vi "FOCUS_V42_H37.vi"(9 "X-pixels":sgl=256.0, 11 "Run":bool) -> (0 "Retrace pixels":sgl, 10 "Pixel Clock (Hz)":sgl)   [LabVIEW 2010] (continued)
                    n2567 = local read "stop 2"() -> (w4781:bool)
                    n2568 = Increment(x=w4763) -> (x+1=w4798:i32)
                    "#" <- w4798
                    n2569 = local read "Overlay Images"() -> (w4802:bool)
                    n2570 = Array Subset "Extract DI0"(array=w4764, index=w4789, length=w4791) -> (w4794:u32[])
                    n2571 = Equal?(x=w4798, y=w4777) -> (x = y?=w4779:bool)
                    n2572 = Split Number(x=w4794) -> (hi(x)=w4753:u16[], lo(x)=w4761:u16[])
                    n2573 = case shown="0, Default" w4760 {
                      tunnel: w4753 -> [w4829 w4834 w4839 w4844 w4849 w4854]
                      tunnel: [w4828 w4833 w4836 w4843 w4848 w4851] -> w4758
                      tunnel: [w4826 w4831 w4838 w4841 w4846 w4853] -> w4757
                      tunnel: w4761 -> [w4827 w4832 w4837 w4842 w4847 w4852]
                      tunnel: [w4825 w4830 w4835 w4840 w4845 w4850] -> w4759
                      frame 0, Default {
                        n2574 = Split Number(x=w4829) -> (hi(x)=w4828:u8[], lo(x)=w4826:u8[])
                        n2575 = Split Number(x=w4827) -> (lo(x)=w4825:u8[])  [unwired: 1 out]
                      }
                      frame 1 {
                        n2576 = Split Number(x=w4834) -> (hi(x)=w4833:u8[], lo(x)=w4830:u8[])
                        n2577 = Split Number(x=w4832) -> (lo(x)=w4831:u8[])  [unwired: 1 out]
                      }
                      frame 2 {
                        n2578 = Split Number(x=w4839) -> (hi(x)=w4835:u8[], lo(x)=w4838:u8[])
                        n2579 = Split Number(x=w4837) -> (lo(x)=w4836:u8[])  [unwired: 1 out]
                      }
                      frame 3 {
                        n2580 = Split Number(x=w4844) -> (hi(x)=w4843:u8[], lo(x)=w4841:u8[])
                        n2581 = Split Number(x=w4842) -> (lo(x)=w4840:u8[])  [unwired: 1 out]
                      }
                      frame 4 {
                        n2582 = Split Number(x=w4849) -> (hi(x)=w4848:u8[], lo(x)=w4845:u8[])
                        n2583 = Split Number(x=w4847) -> (lo(x)=w4846:u8[])  [unwired: 1 out]
                      }
                      frame 5 {
                        n2584 = Split Number(x=w4854) -> (hi(x)=w4850:u8[], lo(x)=w4853:u8[])
                        n2585 = Split Number(x=w4852) -> (lo(x)=w4851:u8[])  [unwired: 1 out]
                      }
                    }
                    n2586 = Set File Position(refnum=w4775, from (0:start)=enum16{"start", "end", "current"}."current" ("pos mode (0:2)"), error in=w4774) -> (refnum out=w4750:refnum<file>, error out=w4749:errorcluster)  [unwired: 1 in]
                    n2587 = Compound Arithmetic op=OR(w4779, w4780, w4781, w4783, w4782, w4784, w4785) -> (w4778:bool)
                    n2588 = Tick Count (ms)() -> (millisecond timer value=w4810:u32)
                    n2589 = case shown="1" w4762 {
                      tunnel: w4758 -> [w4857 w4865]
                      tunnel: [w4857 w4864] -> w4756
                      tunnel: w4763 -> [_ w4860]
                      tunnel: w4757 -> [w4856 w4862]
                      tunnel: [w4856 w4861] -> w4755
                      tunnel: w4759 -> [w4855 w4859]
                      tunnel: [w4855 w4858] -> w4754
                      frame 0, Default {
                      }
                      frame 1 {
                        n2590 = local read "Shift"() -> (w4863:sgl)
                        n2591 = call "testoddevenFOCUS.vi"("Numeric"=w4860) -> ("Boolean"=w4866:bool)
                        n2592 = case shown="True" w4866 {
                          tunnel: w4865 -> [w4869 w4896]
                          tunnel: [w4869 w4898] -> w4864
                          tunnel: w4863 -> [_ w4872]
                          tunnel: w4862 -> [w4868 w4884]
                          tunnel: [w4868 w4883] -> w4861
                          tunnel: w4859 -> [w4867 w4871]
                          tunnel: [w4867 w4870] -> w4858
                          frame False {
                          }
                          frame True {
                            n2593 = Round Toward -Infinity(1:w4872) -> (0:w4888:sgl)
                            n2594 = Round Toward -Infinity(1:w4872) -> (0:w4879:sgl)
                            n2595 = Round Toward -Infinity(1:w4872) -> (0:w4903:sgl)
                            n2596 = To Word Integer(number=w4884) -> (16bit integer=w4894:i16[])
                            n2597 = To Word Integer(number=w4871) -> (16bit integer=w4873:i16[])
                            n2598 = To Word Integer(number=w4896) -> (16bit integer=w4895:i16[])
                            n2599 = Array Subset(array=w4894, index=1) -> (w4887:i16[])  [unwired: 1 in]
                            n2600 = Array Subset(array=w4873, index=1) -> (w4880:i16[])  [unwired: 1 in]
                            n2601 = Array Subset(array=w4895, index=1) -> (w4904:i16[])  [unwired: 1 in]
                            n2602 = Subtract(x=w4872, y=w4888) -> (x-y=w4889:sgl)
                            n2603 = Subtract(x=w4872, y=w4879) -> (x-y=w4878:sgl)
                            n2604 = Subtract(x=w4872, y=w4903) -> (x-y=w4902:sgl)
                            n2605 = Subtract(x=w4894, y=w4887) -> (x-y=w4891:i16[])
                            n2606 = Subtract(x=w4873, y=w4880) -> (x-y=w4876:i16[])
                            n2607 = Subtract(x=w4895, y=w4904) -> (x-y=w4900:i16[])
                            n2608 = Build Array (concatenate)(0 ("index"), w4891) -> (w4892:i32[])
                            n2609 = Build Array (concatenate)(0 ("index"), w4876) -> (w4875:i32[])
                            n2610 = Build Array (concatenate)(0 ("index"), w4900) -> (w4899:i32[])
                            n2611 = Multiply(x=w4889, y=w4892) -> (x*y=w4890:sgl[])
                            n2612 = Multiply(x=w4878, y=w4875) -> (x*y=w4877:sgl[])
                            n2613 = Multiply(x=w4902, y=w4899) -> (x*y=w4901:sgl[])
                            n2614 = Add(x=w4894, y=w4890) -> (x+y=w4885:sgl[])
                            n2615 = To Unsigned Byte Integer(number=w4885) -> (unsigned 8bit integer=w4883:u8[])
                            n2616 = Add(x=w4873, y=w4877) -> (x+y=w4882:sgl[])
                            n2617 = To Unsigned Byte Integer(number=w4882) -> (unsigned 8bit integer=w4870:u8[])
                            n2618 = Add(x=w4895, y=w4901) -> (x+y=w4906:sgl[])
                            n2619 = To Unsigned Byte Integer(number=w4906) -> (unsigned 8bit integer=w4898:u8[])
                          }
                        }
                      }
                    }
                    n2620 = case shown="True" w4802 {
                      tunnel: w4756 -> [w4926 w4929]
                      tunnel: [w4926 w4927] -> w4804
                      tunnel: w4755 -> [w4925 w4928]
                      tunnel: [w4925 _] -> w4803
                      frame False {
                      }
                      frame True {
                        n2621 = To Word Integer(number=w4929) -> (16bit integer=w4934:i16[])
                        n2622 = Subtract(x=w4934, y=w4928) -> (x-y=w4935:i16[])
                        n2623 = Add(x=w4934, y=w4928) -> (x+y=w4939:i16[])
                        n2624 = Increment(x=w4939) -> (x+1=w4930:i16[])
                        n2625 = Divide(x=w4935, y=w4930) -> (x/y=w4931:dbl[])
                        n2626 = Absolute Value(x=w4935) -> (abs(x)=w4937:i16[])
                        n2627 = Multiply(x=w4931, y=u8 2) -> (x*y=w4933:dbl[])
                        n2628 = Round To Nearest(number=w4933) -> (nearest integer value=w4946:dbl[])
                        n2629 = Divide(x=w4937, y=2.0) -> (x/y=w4940:dbl[])
                        n2630 = Divide(x=w4939, y=2.0) -> (x/y=w4941:dbl[])
                        n2631 = Add(x=w4940, y=w4941) -> (x+y=w4943:dbl[])
                        n2632 = Divide(x=w4943, y=5.0) -> (x/y=w4944:dbl[])
                        n2633 = Round To Nearest(number=w4944) -> (nearest integer value=w4945:dbl[])
                        n2634 = Multiply(x=5.0 ("y"), y=w4945) -> (x*y=w4947:dbl[])
                        n2635 = Add(x=w4946, y=w4947) -> (x+y=w4948:dbl[])
                        n2636 = Subtract(x=w4948, y=2.0) -> (x-y=w4951:dbl[])
                        n2637 = To Unsigned Byte Integer(number=w4951) -> (unsigned 8bit integer=w4927:u8[])
                      }
                    }
                    n2638 = Subtract(x=w4763, y=w4791) -> (x-y=w4792:sgl)
                    n2639 = Subtract(x=w4810, y=w4809) -> (x-y=w4811:u32)
                    n2640 = local read "Image Update [ms]"() -> (w4793:u32)
                    n2641 = property class="DAQmx Read"(reference=w4771, error in=w4769) -> (reference out=w4770:refnum<k21>, error out=w4768:errorcluster, "Status:Available Samples Per Channel"=w4767:u32)
                    n2642 = Greater Or Equal?(x=w4811, y=w4793) -> (x >= y?=w4812:bool)
                    n2643 = local write "Scan Backlock"(w4767) -> ()
                    n2644 = case shown="True" w4751 {
                      tunnel: w4756 -> [w4821 w4824]
                      tunnel: w4755 -> [w4818 w4823]
                      tunnel: w4754 -> [w4820 _]
                      tunnel: [w4819 w4822] -> w4752
                      frame True {
                        n2645 = Interleave 1D Arrays(w4818, w4821, w4820) -> (w4819:u8[])
                      }
                      frame False {
                        n2646 = Interleave 1D Arrays(w4824, w4823) -> (w4822:u8[])
                      }
                    }
                    n2647 = Write to Binary File(file (use dialog)=w4750, data=w4752, error in=w4749, 5:FALSE ("prepend array or string size? (T)")) -> (refnum out=w4773:refnum<file>, error out=w4772:errorcluster)  [unwired: 2 in, 1 out]
                    n2648 = local read "X-pixels"() -> (w4813:sgl)
                    n2649 = Subtract(x=w4763, y=w4813) -> (x-y=w4805:sgl)
                    n2650 = Replace Array Subset(array=w4817, new element=w4804, index (col)=w4763) -> (w4815:u8[][])  [unwired: 1 in]
                    n2651 = Replace Array Subset(array=w4816, new element=w4803, index (col)=w4763) -> (w4814:u8[][])  [unwired: 1 in]
                    n2652 = Array Subset(array=w4815, index (col)=w4805, length (col)=w4813) -> (w4807:u8[][])  [unwired: 2 in]
                    n2653 = Array Subset(array=w4814, index (col)=w4805, length (col)=w4813) -> (w4806:u8[][])  [unwired: 2 in]
                    n2654 = case shown="True" w4812 {
                      tunnel: [w4952 w4955] -> w4808
                      tunnel: w4809 -> [w4952 _]
                      tunnel: w4807 -> [_ w4954]
                      tunnel: w4806 -> [_ w4953]
                      frame False {
                      }
                      frame True {
                        n2655 = local write "Image 2"(w4953) -> ()
                        n2656 = local write "Image 1"(w4954) -> ()
                        n2657 = Tick Count (ms)() -> (millisecond timer value=w4955:u32)
                      }
                    }
                  }
                  n2658 = Close File(refnum=w4699, error in=w4700) -> ()  [unwired: 2 out]
                  n2659 = flat-sequence {
                    tunnel: w4732 -> [w4746]
                    tunnel: [w4746] -> w4731
                    frame #0 {
                      n2660 = Tick Count (ms)() -> (millisecond timer value=w4747:u32)
                      n2661 = local write "stop"(w4747) -> ()
                    }
                  }
                }
                frame 3 {
                  w5005 = 0.0 ("X Scale.Range:Minimum")
                  w5018 = 0.0 ("x offset")
                  w5019 = 1.0 ("x offset")
                  w5007 = TRUE ("Visible")
                  # "User-defined line"
                  n2662 = property on="Property Node" class="VI"() -> ("VI Path"=w4973:path)  [unwired: 2 in, 2 out]
                  n2663 = flat-sequence {
                    tunnel: w5012 -> [w5034]
                    tunnel: [w5034] -> w5011
                    frame #0 {
                      n2664 = Tick Count (ms)() -> (millisecond timer value=w5035:u32)
                      n2665 = local write "start"(w5035) -> ()
                    }
                  }
                  n2666 = Greater Or Equal?(x=w4961, y=u16 3) -> (x >= y?=w4959:bool)
                  n2667 = Strip Path(path=w4973) -> (stripped path=w4972:path)  [unwired: 1 out]
                  n2668 = Tick Count (ms)() -> (millisecond timer value=w5025:u32)
                  n2669 = Bundle("x offset"=w5019, "x offset"=w5019, "x offset"=w5018, "x offset"=w5018) -> (w5017:T33)  [unwired: 1 in]
                  n2670 = Build Path(base path=w4972, name or relative path="FreeLine.tmp") -> (appended path=w4971:path)
                  n2671 = Unbundle By Name(w4987) -> ("status"=w4986:bool)
                  n2672 = call <vilib>:"Open_Create_Replace File.vi"("advisory dialog? (display:T)"=FALSE, "function (open:0)"=T8."create or replace", "file path"=w4971) -> ("error out"=w4965:errorcluster, "refnum"=w4967:refnum<file>)  [unwired: 5 in, 2 out]
                  n2673 = Set File Position(refnum=w4967, from (0:start)=enum16{"start", "end", "current"}."start" ("pos mode (rel. to end:1)"), error in=w4965) -> (refnum out=w4958:refnum<file>, error out=w4957:errorcluster)  [unwired: 1 in]
                  n2674 = Write to Binary File(file (use dialog)=w4958, data=w4963, error in=w4957, 5:FALSE ("prepend array or string size? (T)")) -> (refnum out=w4966:refnum<file>, error out=w4964:errorcluster)  [unwired: 2 in, 1 out]
                  n2675 = while {
                    tunnel: [w5055] -> w5026
                    tunnel: [w5056] -> w5010
                    tunnel: w5027 -> [w5101]
                    tunnel: w5011 -> [w5100]
                    shift-right: [w5116] -> w4979
                    shift-left: w5028 -> [w5142]
                    tunnel: w4989 -> [w5098]
                    shift-right: [w5117] -> w4978
                    shift-left: w5028 -> [w5141]
                    shift-right: [w5135] -> _
                    shift-left: w5025 -> [w5136]
                    tunnel: w5023 -> [w5127]
                    tunnel: w5022 -> [w5091]
                    tunnel: [w5126] -> w5021
                    tunnel: [w5125] -> w5020
                    shift-right: [w5122] -> _
                    shift-left: w5017 -> [w5129]
                    tunnel: w5016 -> [w5104]
                    tunnel: w5015 -> [w5092]
                    tunnel: [w5103] -> w5014
                    tunnel: [w5102] -> w5013
                    shift-right: [w5107] -> w4969
                    shift-left: w5003 -> [w5109]
                    tunnel: w4993 -> [w5105]
                    tunnel: w4992 -> [w5083]
                    tunnel: [w5105] -> w4991
                    tunnel: [w5083] -> w4990
                    tunnel: [w5095] -> w4988
                    tunnel: w4986 -> [w5090]
                    shift-right: [w5059] -> w4977
                    shift-left: w4966 -> [w5062]
                    shift-right: [w5060] -> w4976
                    shift-left: w4964 -> [w5061]
                    tunnel: w4962 -> [w5053]
                    tunnel: w4961 -> [w5045]
                    tunnel: w4959 -> [w5039]
                    i -> [w5094]
                    stop <- w5081 stop-if-true
                    # "DIO Read reads one\nline of data at a time"
                    n2676 = Equal To 0?(x=w5094) -> (x = 0?=w5113:bool)
                    n2677 = local read "End experiment"() -> (w5088:bool)
                    n2678 = case shown="True" w5113 {
                      tunnel: w5098 -> [w5208 w5211]
                      tunnel: [w5208 w5210] -> w5050
                      tunnel: w5053 -> [_ w5209]
                      tunnel: [sgl 0.0 w5209] -> w5049
                      frame False {
                      }
                      frame True {
                        n2679 = Add(x=w5211, y=w5209) -> (x+y=w5210:sgl)
                      }
                    }
                    n2680 = call-poly <vilib>:"DAQmx Read (Digital 1D U32 1Chan NSamp).vi"("task/channels in"=w5101, "number of samples per channel"=w5050, "error in"=w5100) -> ("task out"=w5058:refnum<k21>, "data"=w5052:u32[], "error out"=w5057:errorcluster)  [unwired: 10 in]
                    n2681 = Increment(x=w5094) -> (x+1=w5106:i32)
                    "#" <- w5106
                    n2682 = call-poly <vilib>:"DAQmx Read (Analog 2D DBL NChan NSamp).vi"("task/channels in"=w5104, "number of samples per channel"=w5050, "error in"=w5092) -> ("task out"=w5103:refnum<k21>, "data"=w5048:dbl[][], "error out"=w5102:errorcluster)  [unwired: 10 in]
                    n2683 = Unbundle By Name(w5092) -> ("status"=w5082:bool)
                    n2684 = local read "stop 2"() -> (w5089:bool)
                    n2685 = local read "Overlay Images"() -> (w5110:bool)
                    n2686 = Array Subset(array=w5048, index (col)=w5049) -> (w5047:dbl[][])  [unwired: 3 in]
                    n2687 = Unbundle By Name(w5091) -> ("status"=w5084:bool)
                    n2688 = Equal?(x=w5106, y="Y-lines FreeLine") -> (x = y?=w5087:bool)
                    n2689 = Transpose 2D Array(2D array=w5047) -> (transposed array=w5099:dbl[][])
                    n2690 = Unbundle By Name(w5057) -> ("status"=w5085:bool)
                    n2691 = Array Subset "Extract DI0"(array=w5052, index=w5049) -> (w5051:u32[])  [unwired: 1 in]
                    n2692 = Unbundle By Name(w5083) -> ("status"=w5086:bool)
                    n2693 = Split Number(x=w5051) -> (hi(x)=w5041:u16[], lo(x)=w5046:u16[])
                    n2694 = Build Array (concatenate)(w5109, w5099) -> (w5108:dbl[][])
                    n2695 = Index Array(array=w5099, index (col)=0 ("disabled index (col)")) -> (element=w5119:dbl[])  [unwired: 1 in]
                    n2696 = Bundle("x offset"="x offset", "x scale"="x scale", "y offset"="y offset", "y scale"="y scale") -> (w5122:T34)  [unwired: 1 in]
                    n2697 = Array Subset(array=w5108, index (row)=w5098) -> (w5107:dbl[][])  [unwired: 3 in]
                    n2698 = Index Array(array=w5099, index (col)=1 ("disabled index (col)")) -> (element=w5118:dbl[])  [unwired: 1 in]
                    n2699 = Tick Count (ms)() -> (millisecond timer value=w5137:u32)
                    n2700 = Not Equal?(x=w5129, y=w5122) -> (x != y?=w5128:bool)
                    n2701 = Compound Arithmetic op=OR(w5082, w5084, w5085, w5086, w5087, w5088, w5089, w5090) -> (w5081:bool)
                    n2702 = case shown="True" w5128 {
                      tunnel: w5127 -> [w5213 w5218]
                      tunnel: w5091 -> [w5212 w5215]
                      tunnel: [w5213 w5216] -> w5126
                      tunnel: [w5212 w5214] -> w5125
                      tunnel: w5122 -> [_ w5220]
                      frame False {
                      }
                      frame True {
                        n2703 = local read "ScanLineFreeLine"() -> (w5219:sgl[][])
                        n2704 = call "ScaleudlFOCUS.vi"("Cluster"=w5220, "ScanLineUDL"=w5219) -> ("ScanLineUDLnew"=w5217:dbl[][])
                        n2705 = call-poly <vilib>:"DAQmx Write (Analog 2D DBL NChan NSamp).vi"("task/channels in"=w5218, "data"=w5217, "error in"=w5215) -> ("task out"=w5216:refnum<k21>, "error out"=w5214:errorcluster)  [unwired: 10 in, 1 out]
                      }
                    }
                    n2706 = case shown="0, Default" w5045 {
                      tunnel: w5041 -> [w5154 w5159 w5164 w5169 w5174 w5179]
                      tunnel: [w5153 w5158 w5161 w5168 w5173 w5176] -> w5042
                      tunnel: [w5151 w5156 w5163 w5166 w5171 w5178] -> w5043
                      tunnel: w5046 -> [w5152 w5157 w5162 w5167 w5172 w5177]
                      tunnel: [w5150 w5155 w5160 w5165 w5170 w5175] -> w5044
                      frame 0, Default {
                        n2707 = Split Number(x=w5154) -> (hi(x)=w5153:u8[], lo(x)=w5151:u8[])
                        n2708 = Split Number(x=w5152) -> (lo(x)=w5150:u8[])  [unwired: 1 out]
                      }
                      frame 1 {
                        n2709 = Split Number(x=w5159) -> (hi(x)=w5158:u8[], lo(x)=w5155:u8[])
                        n2710 = Split Number(x=w5157) -> (lo(x)=w5156:u8[])  [unwired: 1 out]
                      }
                      frame 2 {
                        n2711 = Split Number(x=w5164) -> (hi(x)=w5160:u8[], lo(x)=w5163:u8[])
                        n2712 = Split Number(x=w5162) -> (lo(x)=w5161:u8[])  [unwired: 1 out]
                      }
                      frame 3 {
                        n2713 = Split Number(x=w5169) -> (hi(x)=w5168:u8[], lo(x)=w5166:u8[])
                        n2714 = Split Number(x=w5167) -> (lo(x)=w5165:u8[])  [unwired: 1 out]
                      }
                      frame 4 {
                        n2715 = Split Number(x=w5174) -> (hi(x)=w5173:u8[], lo(x)=w5170:u8[])
                        n2716 = Split Number(x=w5172) -> (lo(x)=w5171:u8[])  [unwired: 1 out]
                      }
                      frame 5 {
                        n2717 = Split Number(x=w5179) -> (hi(x)=w5175:u8[], lo(x)=w5178:u8[])
                        n2718 = Split Number(x=w5177) -> (lo(x)=w5176:u8[])  [unwired: 1 out]
                      }
                    }
                    n2719 = case shown="True" w5110 {
                      tunnel: w5042 -> [w5181 w5184]
                      tunnel: [w5181 w5182] -> w5112
                      tunnel: w5043 -> [w5180 w5183]
                      tunnel: [w5180 _] -> w5111
                      frame False {
                      }
                      frame True {
                        n2720 = To Word Integer(number=w5184) -> (16bit integer=w5189:i16[])
                        n2721 = Subtract(x=w5189, y=w5183) -> (x-y=w5190:i16[])
                        n2722 = Add(x=w5189, y=w5183) -> (x+y=w5194:i16[])
                        n2723 = Increment(x=w5194) -> (x+1=w5185:i16[])
                        n2724 = Divide(x=w5190, y=w5185) -> (x/y=w5186:dbl[])
                        n2725 = Absolute Value(x=w5190) -> (abs(x)=w5192:i16[])
                        n2726 = Multiply(x=w5186, y=u8 2) -> (x*y=w5188:dbl[])
                        n2727 = Round To Nearest(number=w5188) -> (nearest integer value=w5201:dbl[])
                        n2728 = Divide(x=w5192, y=2.0) -> (x/y=w5195:dbl[])
                        n2729 = Divide(x=w5194, y=2.0) -> (x/y=w5196:dbl[])
                        n2730 = Add(x=w5195, y=w5196) -> (x+y=w5198:dbl[])
                        n2731 = Divide(x=w5198, y=5.0) -> (x/y=w5199:dbl[])
                        n2732 = Round To Nearest(number=w5199) -> (nearest integer value=w5200:dbl[])
                        n2733 = Multiply(x=5.0 ("y"), y=w5200) -> (x*y=w5202:dbl[])
                        n2734 = Add(x=w5201, y=w5202) -> (x+y=w5203:dbl[])
                        n2735 = Subtract(x=w5203, y=2.0) -> (x-y=w5206:dbl[])
                        n2736 = To Unsigned Byte Integer(number=w5206) -> (unsigned 8bit integer=w5182:u8[])
                      }
                    }
                    n2737 = Subtract(x=w5137, y=w5136) -> (x-y=w5138:u32)
                    n2738 = local read "Image Update [ms]"() -> (w5097:u32)
                    n2739 = property class="DAQmx Read"(reference=w5058, error in=w5057) -> (reference out=w5055:refnum<k21>, error out=w5056:errorcluster, "Status:Available Samples Per Channel"=w5054:u32)
                    n2740 = Multiply(x="x scale", y=w5119) -> (x*y=w5133:dbl[])
                    n2741 = Greater Or Equal?(x=w5138, y=w5097) -> (x >= y?=w5139:bool)
                    n2742 = Multiply(x=w5118, y="y scale") -> (x*y=w5132:dbl[])
                    n2743 = case shown="True" w5039 {
                      tunnel: w5042 -> [w5146 w5149]
                      tunnel: w5043 -> [w5143 w5148]
                      tunnel: w5044 -> [w5145 _]
                      tunnel: [w5144 w5147] -> w5040
                      frame True {
                        n2744 = Interleave 1D Arrays(w5143, w5146, w5145) -> (w5144:u8[])
                      }
                      frame False {
                        n2745 = Interleave 1D Arrays(w5149, w5148) -> (w5147:u8[])
                      }
                    }
                    n2746 = Add(x="x offset", y=w5133) -> (x+y=w5065:dbl[])
                    n2747 = Add(x=w5132, y="y offset") -> (x+y=w5067:dbl[])
                    n2748 = local write "Scan Backlock"(w5054) -> ()
                    n2749 = local read "y jog"() -> (w5068:sgl)
                    n2750 = local read "x jog"() -> (w5069:sgl)
                    n2751 = Subtract(x=w5067, y=w5068) -> (x-y=w5066:dbl[])
                    n2752 = Subtract(x=w5065, y=w5069) -> (x-y=w5064:dbl[])
                    n2753 = local read "Zoom"() -> (w5070:sgl)
                    n2754 = local read "X-pixels FreeLine"() -> (w5096:sgl)
                    n2755 = Replace Array Subset(array=w5142, new element=w5112, index (col)=w5094) -> (w5116:u8[][])  [unwired: 1 in]
                    n2756 = Replace Array Subset(array=w5141, new element=w5111, index (col)=w5094) -> (w5117:u8[][])  [unwired: 1 in]
                    n2757 = Multiply(x=w5066, y=w5070) -> (x*y=w5072:dbl[])
                    n2758 = Multiply(x=w5064, y=w5070) -> (x*y=w5071:dbl[])
                    n2759 = Subtract(x=w5094, y=w5096) -> (x-y=w5140:sgl)
                    n2760 = Set File Position(refnum=w5062, from (0:start)=enum16{"start", "end", "current"}."current" ("pos mode (0:2)"), error in=w5061) -> (refnum out=w5038:refnum<file>, error out=w5037:errorcluster)  [unwired: 1 in]
                    n2761 = Write to Binary File(file (use dialog)=w5038, data=w5040, error in=w5037, 5:FALSE ("prepend array or string size? (T)")) -> (refnum out=w5059:refnum<file>, error out=w5060:errorcluster)  [unwired: 2 in, 1 out]
                    n2762 = Array Subset(array=w5116, index (col)=w5140, length (col)=w5096) -> (w5115:u8[][])  [unwired: 2 in]
                    n2763 = Multiply(x=sgl -2.7 ("X Factor"), y=w5072) -> (x*y=w5078:dbl[])
                    n2764 = Multiply(x=sgl -2.7 ("X Factor"), y=w5071) -> (x*y=w5074:dbl[])
                    n2765 = Subtract(x=w5094, y=w5096) -> (x-y=w5095:sgl)
                    n2766 = Array Subset(array=w5117, index (col)=w5140, length (col)=w5096) -> (w5114:u8[][])  [unwired: 2 in]
                    n2767 = Add(x=sgl -0.005 ("X Offset"), y=w5078) -> (x+y=w5077:dbl[])
                    n2768 = Add(x=sgl -0.025 ("X Offset"), y=w5074) -> (x+y=w5073:dbl[])
                    n2769 = Bundle(w5073, w5077) -> (w5134:cluster{dbl[], dbl[]})  [unwired: 1 in]
                    n2770 = case shown="True" w5139 {
                      tunnel: [w5221 w5225] -> w5135
                      tunnel: w5136 -> [w5221 _]
                      tunnel: w5134 -> [_ w5224]
                      tunnel: w5115 -> [_ w5223]
                      tunnel: w5114 -> [_ w5222]
                      frame False {
                      }
                      frame True {
                        n2771 = local write "XY Graph 3"(w5224) -> ()
                        n2772 = local write "XY Graph 4"(w5224) -> ()
                        n2773 = local write "Image 4"(w5222) -> ()
                        n2774 = local write "Image 3"(w5223) -> ()
                        n2775 = Tick Count (ms)() -> (millisecond timer value=w5225:u32)
                      }
                    }
                  }
                  n2776 = local read "X-pixels FreeLine"() -> (w5008:sgl)
                  n2777 = property on="Image 2" class="IntGraph (strict)"() -> ("Color Table"=w5006:u32[])  [unwired: 2 in, 2 out]
                  n2778 = Decrement(x=w5008) -> (x-1=w5004:sgl)
                  n2779 = property on="Image 3" class="IntGraph (strict)"("X Scale.Range:Minimum"=w5005, "X Scale.Range:Maximum"=w5004, "Y Scale.Range:Minimum"=w5005, "Y Scale.Range:Maximum"=w5004, "Visible"=w5007, "Color Table"=w5006) -> ()  [unwired: 2 in, 2 out]
                  n2780 = property on="Image 4" class="IntGraph (strict)"("X Scale.Range:Minimum"=w5005, "X Scale.Range:Maximum"=w5004, "Y Scale.Range:Minimum"=w5005, "Y Scale.Range:Maximum"=w5004, "Visible"=w5007, "Color Table"=w5006) -> ()  [unwired: 2 in, 2 out]
                  n2781 = property on="Histogram1" class="XYGraph (strict)"("X Scale.Range:Minimum"=w5005, "X Scale.Range:Maximum"=w5004) -> ()  [unwired: 2 in, 2 out]
                  n2782 = property on="Histogram2" class="XYGraph (strict)"("X Scale.Range:Minimum"=w5005, "X Scale.Range:Maximum"=w5004) -> ()  [unwired: 2 in, 2 out]
                  n2783 = Close File(refnum=w4977, error in=w4976) -> ()  [unwired: 2 out]
                  n2784 = Array Subset(array=w4969, index (col)=0 ("index"), length (col)=3 ("length")) -> (w4994:dbl[][])  [unwired: 2 in]
                  n2785 = Index Array(array=w4994, index (col)=0 ("disabled index (col)")) -> (element=w5001:dbl[])  [unwired: 1 in]
                  n2786 = Array Size(array=w5001) -> (size(s)=w5000:i32)
                  n2787 = Multiply(x=w5000, y=3) -> (x*y=w4998:i32)
                  n2788 = Reshape Array(w4994, w4998) -> (→"Positions":dbl[])
                  n2789 = flat-sequence {
                    tunnel: [w5032] -> w5009
                    tunnel: w5010 -> [w5032]
                    frame #0 {
                      n2790 = Tick Count (ms)() -> (millisecond timer value=w5033:u32)
                      n2791 = local write "stop"(w5033) -> ()
                    }
                  }
                }
                frame 4 {
                  # "Iinner while loop runs for n loops, where n = number of averages.\nAll data acquired in this loop enters the average.\nThe z-step is activated each time this loop completes..\nThe outer while loop iterates m times, where m is total number of frames.\nControls are reset after the outer while loop completes.\nThe shutter is closed before and opened after each z-step."
                  # "Frame scan piezo"
                  n2792 = local read "z-step (um)"() -> (w5231:sgl)
                  n2793 = flat-sequence {
                    tunnel: w5288 -> [w5305]
                    tunnel: [w5305] -> w5287
                    frame #0 {
                      n2794 = Tick Count (ms)() -> (millisecond timer value=w5306:u32)
                      n2795 = local write "start"(w5306) -> ()
                    }
                  }
                  n2796 = local read "Number of frames"() -> (w5289:sgl)
                  n2797 = Unbundle By Name(w5258) -> ("status"=w5257:bool)
                  n2798 = local read "z-step (um)"() -> (w5296:sgl)
                  n2799 = property on="Property Node" class="VI"() -> ("VI Path"=w5245:path)  [unwired: 2 in, 2 out]
                  n2800 = Initialize Array(u8 0 ("element"), w5272, w5273) -> (w5285:u8[][])
                  n2801 = Equal To 0?(x=w5231) -> (x = 0?=w5230:bool)
                  n2802 = Initialize Array(0.0 ("element"), 0 ("dimension size")) -> (w5295:dbl[])
                  n2803 = Strip Path(path=w5245) -> (stripped path=w5244:path)  [unwired: 1 out]
                  n2804 = while {
                    tunnel: w5296 -> [w5317]
                    shift-right: [w5315] -> w5291
                    shift-left: w5295 -> [w5316]
                    tunnel: w5289 -> [w5309]
                    i -> [w5308]
                    stop <- w5310 stop-if-true
                    n2805 = Multiply(x=w5317, y=w5308) -> (x*y=w5313:sgl)
                    n2806 = Increment(x=w5308) -> (x+1=w5307:i32)
                    n2807 = Build Array (concatenate)(w5316, w5313) -> (w5315:dbl[])
                    n2808 = Greater Or Equal?(x=w5313, y=400.0) -> (x >= y?=w5311:bool)
                    n2809 = Greater Or Equal?(x=w5307, y=w5309) -> (x >= y?=w5312:bool)
                    n2810 = Or(x=w5311, y=w5312) -> (x .or. y?=w5310:bool)
                  }
                  n2811 = Build Path(base path=w5244, name or relative path="Stack.tmp") -> (appended path=w5243:path)
                  n2812 = call <vilib>:"Open_Create_Replace File.vi"("advisory dialog? (display:T)"=FALSE, "function (open:0)"=T8."create or replace", "file path"=w5243) -> ("error out"=w5236:errorcluster, "refnum"=w5238:refnum<file>)  [unwired: 5 in, 2 out]
                  n2813 = Divide(x=w5291, y=40.0) -> (x/y=w5269:dbl[])
                  n2814 = Set File Position(refnum=w5238, from (0:start)=enum16{"start", "end", "current"}."start" ("pos mode (rel. to end:1)"), error in=w5236) -> (refnum out=w5228:refnum<file>, error out=w5227:errorcluster)  [unwired: 1 in]
                  n2815 = Write to Binary File(file (use dialog)=w5228, data=w5234, error in=w5227, 5:FALSE ("prepend array or string size? (T)")) -> (refnum out=w5237:refnum<file>, error out=w5235:errorcluster)  [unwired: 2 in, 1 out]
                  n2816 = Array Subset(array=w5269, index=1) -> (w5268:dbl[])  [unwired: 1 in]
                  n2817 = local read "IntensityAutomatic"() -> (w5253:bool)
                  n2818 = local read "Intensity"() -> (w5255:sgl)
                  n2819 = while {
                    tunnel: [w5393] -> w5267
                    tunnel: [w5392] -> w5266
                    tunnel: w5301 -> [w5391]
                    tunnel: w5287 -> [w5350]
                    tunnel: w5300 -> [w5326]
                    tunnel: w5290 -> [w5390]
                    tunnel: w5268 -> [w5361] mode=indexing
                    tunnel: w5269 -> [w5389]
                    shift-right: [w5387] -> w5251
                    shift-left: w5285 -> [w5388]
                    shift-right: [w5385] -> w5252
                    shift-left: w5285 -> [w5386]
                    tunnel: w5281 -> [w5384]
                    tunnel: w5280 -> [w5353]
                    tunnel: [w5383] -> w5278
                    tunnel: [w5382] -> w5279
                    tunnel: w5277 -> [w5367]
                    tunnel: w5276 -> [w5366]
                    tunnel: [w5372] -> w5275
                    tunnel: [w5371] -> w5274
                    tunnel: [w5357] -> w5271
                    tunnel: w5261 -> [w5365]
                    tunnel: [w5358] -> w5262
                    tunnel: w5255 -> [w5360]
                    tunnel: w5260 -> [w5356]
                    tunnel: [w5354] -> w5259
                    tunnel: w5257 -> [w5348]
                    tunnel: [w5342] -> w5254
                    tunnel: w5253 -> [w5341]
                    shift-right: [w5337] -> w5241
                    shift-left: w5237 -> [w5339]
                    shift-right: [w5336] -> w5240
                    shift-left: w5235 -> [w5338]
                    tunnel: w5233 -> [w5332]
                    tunnel: w5232 -> [w5323]
                    tunnel: w5230 -> [w5329]
                    tunnel: w5229 -> [w5322]
                    i -> [w5354]
                    stop <- w5328 stop-if-true
                    n2820 = Equal To 0?(x=w5354) -> (x = 0?=w5330:bool)
                    n2821 = Or(x=w5330, y=w5329) -> (x .or. y?=w5331:bool)
                    n2822 = case shown="False" w5331 {
                      tunnel: w5367 -> [w5469 w5478]
                      tunnel: [w5462 w5478] -> w5362
                      tunnel: w5366 -> [w5468 w5479]
                      tunnel: [w5461 w5479] -> w5352
                      tunnel: w5356 -> [w5466 w5476]
                      tunnel: w5365 -> [w5465 w5477]
                      tunnel: [w5460 w5477] -> w5351
                      tunnel: [w5459 w5476] -> w5364
                      frame False {
                        w5467 = TRUE ("data")
                        n2823 = local write "Shutter open"(w5467) -> ()
                        n2824 = call-poly <vilib>:"DAQmx Write (Digital Bool 1Line 1Point).vi"("task/channels in"=w5469, "data"=w5467, "error in"=w5468) -> ("task out"=w5464:refnum<k21>, "error out"=w5463:errorcluster)  [unwired: 10 in, 1 out]
                        n2825 = flat-sequence {
                          tunnel: w5466 -> [w5475]
                          tunnel: w5465 -> [w5474]
                          tunnel: w5464 -> [w5473]
                          tunnel: [w5473] -> w5462
                          tunnel: [w5472] -> w5461
                          tunnel: w5463 -> [w5472]
                          tunnel: [w5471] -> w5460
                          tunnel: [w5470] -> w5459
                          frame #0 {
                            n2826 = call <vilib>:"DAQmx Start Task.vi"("task/channels in"=w5475, "error in"=w5474) -> ("task out"=w5470:refnum<k21>, "error out"=w5471:errorcluster)  [unwired: 12 in]
                          }
                        }
                      }
                      frame True {
                      }
                    }
                    n2827 = Greater Or Equal?(x=w5322, y=u16 3) -> (x >= y?=w5321:bool)
                    n2828 = local read "Number of frames"() -> (w5355:sgl)
                    n2829 = Tick Count (ms)() -> (millisecond timer value=w5374:u32)
                    n2830 = Array Size(array=w5389) -> (size(s)=w5377:i32)
                    n2831 = Unbundle By Name(w5353) -> ("status"=w5349:bool)
                    n2832 = Increment(x=w5354) -> (x+1=w5373:i32)
                    n2833 = Equal?(x=w5355, y=w5373) -> (x = y?=w5375:bool)
                    n2834 = Equal?(x=w5373, y=w5377) -> (x = y?=w5376:bool)
                    n2835 = Compound Arithmetic op=OR(w5349, w5348) -> (w5346:bool)
                    n2836 = while {
                      tunnel: [w5510] -> w5393
                      tunnel: [w5512] -> w5392
                      tunnel: w5391 -> [w5559]
                      tunnel: w5350 -> [w5558]
                      shift-right: [w5545] -> w5335
                      shift-left: w5326 -> [w5546]
                      tunnel: w5390 -> [w5529]
                      shift-right: [w5541] -> w5334
                      shift-left: w5326 -> [w5544]
                      tunnel: [w5517] -> w5345
                      tunnel: [w5518] -> w5344
                      shift-right: [w5562] -> _
                      shift-left: w5374 -> [w5563]
                      tunnel: [w5533] -> w5370
                      tunnel: w5362 -> [w5533]
                      tunnel: [w5523] -> w5368
                      tunnel: w5352 -> [w5523]
                      tunnel: [w5532] -> w5359
                      tunnel: w5364 -> [w5532]
                      tunnel: [w5524] -> w5363
                      tunnel: w5351 -> [w5524]
                      tunnel: w5346 -> [w5516]
                      tunnel: [w5514] -> w5343
                      tunnel: w5332 -> [w5508]
                      tunnel: w5323 -> [w5497]
                      tunnel: w5330 -> [w5504]
                      shift-right: [w5483] -> w5325
                      shift-left: w5326 -> [w5485]
                      tunnel: w5322 -> [w5482]
                      i -> [w5496]
                      stop <- w5515 stop-if-true
                      # "DIO Read reads one\nline of data at a time"
                      n2837 = local read "z-step (um)"() -> (w5506:sgl)
                      n2838 = local read "Scan Cut-Off (either end)"() -> (w5560:sgl)
                      n2839 = local read "End experiment"() -> (w5518:bool)
                      n2840 = Equal To 0?(x=w5496) -> (x = 0?=w5505:bool)
                      n2841 = Equal To 0?(x=w5506) -> (x = 0?=w5507:bool)
                      n2842 = local read "Overlay Images"() -> (w5561:bool)
                      n2843 = Unbundle By Name(w5524) -> ("status"=w5521:bool)
                      n2844 = Unbundle By Name(w5523) -> ("status"=w5520:bool)
                      n2845 = local read "X-pixels"() -> (w5557:sgl)
                      n2846 = local read "Cusp Delay"() -> (w5527:sgl)
                      n2847 = local read "stop 2"() -> (w5517:bool)
                      n2848 = case shown="True" w5507 {
                        tunnel: w5504 -> [_ w5651]
                        tunnel: w5505 -> [w5648 w5650]
                        tunnel: [w5648 w5649] -> w5503
                        frame False {
                        }
                        frame True {
                          n2849 = And(x=w5650, y=w5651) -> (x .and. y?=w5649:bool)
                        }
                      }
                      n2850 = case shown="False" w5503 {
                        tunnel: w5529 -> [w5668 w5673]
                        tunnel: [w5668 w5672] -> w5528
                        tunnel: w5560 -> [w5667 w5671]
                        tunnel: [w5667 w5670] -> w5525
                        tunnel: w5508 -> [_ w5669]
                        frame False {
                        }
                        frame True {
                          n2851 = Add(x=w5673, y=w5669) -> (x+y=w5672:sgl)
                          n2852 = Add(x=w5671, y=w5669) -> (x+y=w5670:sgl)
                        }
                      }
                      n2853 = call-poly <vilib>:"DAQmx Read (Digital 1D U32 1Chan NSamp).vi"("task/channels in"=w5559, "number of samples per channel"=w5528, "error in"=w5558) -> ("task out"=w5511:refnum<k21>, "data"=w5501:u32[], "error out"=w5513:errorcluster)  [unwired: 10 in]
                      n2854 = case shown="1" w5497 {
                        tunnel: w5496 -> [_ w5657]
                        tunnel: w5501 -> [w5652 w5655]
                        tunnel: [w5652 w5654] -> w5500
                        frame 0, Default {
                        }
                        frame 1 {
                          n2855 = local read "Shift"() -> (w5653:sgl)
                          n2856 = call "testoddevenFOCUS.vi"("Numeric"=w5657) -> ("Boolean"=w5656:bool)
                          n2857 = case shown="True" w5656 {
                            tunnel: w5655 -> [w5659 w5662]
                            tunnel: [w5658 w5660] -> w5654
                            tunnel: w5653 -> [_ w5661]
                            frame False {
                              n2858 = Reverse 1D Array(array=w5659) -> (reversed array=w5658:u32[])
                            }
                            frame True {
                              n2859 = Rotate 1D Array(1:w5662, 2:w5661) -> (0:w5660:u32[])
                            }
                          }
                        }
                      }
                      n2860 = Add(x=w5527, y=w5525) -> (x+y=w5526:sgl)
                      n2861 = Array Subset "Extract DI0"(array=w5500, index=w5526, length=w5557) -> (w5502:u32[])
                      n2862 = Split Number(x=w5502) -> (hi(x)=w5495:u16[], lo(x)=w5494:u16[])
                      n2863 = case shown="0, Default" w5482 {
                        tunnel: w5495 -> [w5570 w5575 w5580 w5585 w5590 w5595]
                        tunnel: [w5569 w5574 w5577 w5584 w5589 w5592] -> w5493
                        tunnel: [w5567 w5572 w5579 w5582 w5587 w5594] -> w5492
                        tunnel: w5494 -> [w5568 w5573 w5578 w5583 w5588 w5593]
                        tunnel: [w5566 w5571 w5576 w5581 w5586 w5591] -> w5491
                        frame 0, Default {
                          n2864 = Split Number(x=w5570) -> (hi(x)=w5569:u8[], lo(x)=w5567:u8[])
                          n2865 = Split Number(x=w5568) -> (lo(x)=w5566:u8[])  [unwired: 1 out]
                        }
                        frame 1 {
                          n2866 = Split Number(x=w5575) -> (hi(x)=w5574:u8[], lo(x)=w5571:u8[])
                          n2867 = Split Number(x=w5573) -> (lo(x)=w5572:u8[])  [unwired: 1 out]
                        }
                        frame 2 {
                          n2868 = Split Number(x=w5580) -> (hi(x)=w5576:u8[], lo(x)=w5579:u8[])
                          n2869 = Split Number(x=w5578) -> (lo(x)=w5577:u8[])  [unwired: 1 out]
                        }
                        frame 3 {
                          n2870 = Split Number(x=w5585) -> (hi(x)=w5584:u8[], lo(x)=w5582:u8[])
                          n2871 = Split Number(x=w5583) -> (lo(x)=w5581:u8[])  [unwired: 1 out]
                        }
                        frame 4 {
                          n2872 = Split Number(x=w5590) -> (hi(x)=w5589:u8[], lo(x)=w5586:u8[])
                          n2873 = Split Number(x=w5588) -> (lo(x)=w5587:u8[])  [unwired: 1 out]
                        }
                        frame 5 {
                          n2874 = Split Number(x=w5595) -> (hi(x)=w5591:u8[], lo(x)=w5594:u8[])
                          n2875 = Split Number(x=w5593) -> (lo(x)=w5592:u8[])  [unwired: 1 out]
                        }
                      }
                      n2876 = Unbundle By Name(w5513) -> ("status"=w5522:bool)
                      n2877 = case shown="1" w5497 {
                        tunnel: w5493 -> [w5598 w5605]
                        tunnel: [w5598 w5604] -> w5499
                        tunnel: w5496 -> [_ w5607]
                        tunnel: w5492 -> [w5597 w5602]
                        tunnel: [w5597 w5601] -> w5498
                        tunnel: w5491 -> [w5596 w5600]
                        tunnel: [w5596 w5599] -> w5480
                        frame 0, Default {
                        }
                        frame 1 {
                          n2878 = local read "Shift"() -> (w5603:sgl)
                          n2879 = call "testoddevenFOCUS.vi"("Numeric"=w5607) -> ("Boolean"=w5606:bool)
                          n2880 = case shown="True" w5606 {
                            tunnel: w5605 -> [w5610 w5637]
                            tunnel: [w5610 w5639] -> w5604
                            tunnel: w5603 -> [_ w5613]
                            tunnel: w5602 -> [w5609 w5625]
                            tunnel: [w5609 w5624] -> w5601
                            tunnel: w5600 -> [w5608 w5612]
                            tunnel: [w5608 w5611] -> w5599
                            frame False {
                            }
                            frame True {
                              n2881 = Round Toward -Infinity(1:w5613) -> (0:w5629:sgl)
                              n2882 = Round Toward -Infinity(1:w5613) -> (0:w5644:sgl)
                              n2883 = Round Toward -Infinity(1:w5613) -> (0:w5620:sgl)
                              n2884 = To Word Integer(number=w5625) -> (16bit integer=w5635:i16[])
                              n2885 = To Word Integer(number=w5637) -> (16bit integer=w5636:i16[])
                              n2886 = To Word Integer(number=w5612) -> (16bit integer=w5614:i16[])
                              n2887 = Array Subset(array=w5635, index=1) -> (w5628:i16[])  [unwired: 1 in]
                              n2888 = Array Subset(array=w5636, index=1) -> (w5645:i16[])  [unwired: 1 in]
                              n2889 = Array Subset(array=w5614, index=1) -> (w5621:i16[])  [unwired: 1 in]
                              n2890 = Subtract(x=w5613, y=w5629) -> (x-y=w5630:sgl)
                              n2891 = Subtract(x=w5613, y=w5644) -> (x-y=w5643:sgl)
                              n2892 = Subtract(x=w5613, y=w5620) -> (x-y=w5619:sgl)
                              n2893 = Subtract(x=w5635, y=w5628) -> (x-y=w5632:i16[])
                              n2894 = Subtract(x=w5636, y=w5645) -> (x-y=w5641:i16[])
                              n2895 = Subtract(x=w5614, y=w5621) -> (x-y=w5617:i16[])
                              n2896 = Build Array (concatenate)(0 ("index"), w5632) -> (w5633:i32[])
                              n2897 = Build Array (concatenate)(0 ("index"), w5641) -> (w5640:i32[])
                              n2898 = Build Array (concatenate)(0 ("index"), w5617) -> (w5616:i32[])
                              n2899 = Multiply(x=w5630, y=w5633) -> (x*y=w5631:sgl[])
                              n2900 = Multiply(x=w5643, y=w5640) -> (x*y=w5642:sgl[])
                              n2901 = Multiply(x=w5619, y=w5616) -> (x*y=w5618:sgl[])
                              n2902 = Add(x=w5635, y=w5631) -> (x+y=w5626:sgl[])
                              n2903 = To Unsigned Byte Integer(number=w5626) -> (unsigned 8bit integer=w5624:u8[])
                              n2904 = Add(x=w5636, y=w5642) -> (x+y=w5647:sgl[])
                              n2905 = To Unsigned Byte Integer(number=w5647) -> (unsigned 8bit integer=w5639:u8[])
                              n2906 = Add(x=w5614, y=w5618) -> (x+y=w5623:sgl[])
                              n2907 = To Unsigned Byte Integer(number=w5623) -> (unsigned 8bit integer=w5611:u8[])
                            }
                          }
                        }
                      }
                      n2908 = case shown="True" w5561 {
                        tunnel: w5499 -> [w5675 w5678]
                        tunnel: [w5675 w5676] -> w5543
                        tunnel: w5498 -> [w5674 w5677]
                        tunnel: [w5674 _] -> w5542
                        frame False {
                        }
                        frame True {
                          n2909 = To Word Integer(number=w5678) -> (16bit integer=w5683:i16[])
                          n2910 = Subtract(x=w5683, y=w5677) -> (x-y=w5684:i16[])
                          n2911 = Add(x=w5683, y=w5677) -> (x+y=w5688:i16[])
                          n2912 = Increment(x=w5688) -> (x+1=w5679:i16[])
                          n2913 = Divide(x=w5684, y=w5679) -> (x/y=w5680:dbl[])
                          n2914 = Absolute Value(x=w5684) -> (abs(x)=w5686:i16[])
                          n2915 = Multiply(x=w5680, y=u8 2) -> (x*y=w5682:dbl[])
                          n2916 = Round To Nearest(number=w5682) -> (nearest integer value=w5695:dbl[])
                          n2917 = Divide(x=w5686, y=2.0) -> (x/y=w5689:dbl[])
                          n2918 = Divide(x=w5688, y=2.0) -> (x/y=w5690:dbl[])
                          n2919 = Add(x=w5689, y=w5690) -> (x+y=w5692:dbl[])
                          n2920 = Divide(x=w5692, y=5.0) -> (x/y=w5693:dbl[])
                          n2921 = Round To Nearest(number=w5693) -> (nearest integer value=w5694:dbl[])
                          n2922 = Multiply(x=5.0 ("y"), y=w5694) -> (x*y=w5696:dbl[])
                          n2923 = Add(x=w5695, y=w5696) -> (x+y=w5697:dbl[])
                          n2924 = Subtract(x=w5697, y=2.0) -> (x-y=w5700:dbl[])
                          n2925 = To Unsigned Byte Integer(number=w5700) -> (unsigned 8bit integer=w5676:u8[])
                        }
                      }
                      n2926 = Compound Arithmetic op=OR(w5522, w5521, w5520) -> (w5514:bool)
                      n2927 = property class="DAQmx Read"(reference=w5511, error in=w5513) -> (reference out=w5510:refnum<k21>, error out=w5512:errorcluster, "Status:Available Samples Per Channel"=w5509:u32)
                      n2928 = local read "total y pixels"() -> (w5537:sgl)
                      n2929 = local read "Averaging"() -> (w5540:u16)
                      n2930 = local write "Scan Backlock"(w5509) -> ()
                      n2931 = Multiply(x=w5537, y=w5540) -> (x*y=w5564:sgl)
                      n2932 = Increment(x=w5496) -> (x+1=w5538:i32)
                      n2933 = Equal?(x=w5538, y=w5564) -> (x = y?=w5519:bool)
                      n2934 = Tick Count (ms)() -> (millisecond timer value=w5534:u32)
                      n2935 = Subtract(x=w5534, y=w5563) -> (x-y=w5535:u32)
                      n2936 = Divide(x=w5538, y=w5537) -> (x/y=w5539:sgl)
                      n2937 = local read "Image Update [ms]"() -> (w5531:u32)
                      n2938 = Round Toward +Infinity(x=w5539) -> (ceil(x): smallest int >= x=w5530:sgl)
                      n2939 = Compound Arithmetic op=OR(w5519, w5518, w5517, w5514, w5516) -> (w5515:bool)
                      n2940 = local write "#"(w5530) -> ()
                      n2941 = local read "total y pixels"() -> (w5565:sgl)
                      n2942 = while {
                        tunnel: w5565 -> [w5703]
                        shift-right: [w5704] -> _
                        shift-left: w5496 -> [w5702]
                        tunnel: [w5702] -> w5484
                        tunnel: [w5701] -> w5481
                        i -> [w5701]
                        stop <- w5705 stop-if-true
                        n2943 = Subtract(x=w5702, y=w5703) -> (x-y=w5704:sgl)
                        n2944 = Less?(x=w5702, y=w5703) -> (x < y?=w5705:bool)
                      }
                      n2945 = Index Array(array=w5546, index (col)=w5484) -> (element=w5556:u8[])  [unwired: 1 in]
                      n2946 = Index Array(array=w5485, index (col)=w5484) -> (element=w5486:u8[])  [unwired: 1 in]
                      n2947 = Multiply(x=w5556, y=w5481) -> (x*y=w5555:i32[])
                      n2948 = Greater Or Equal?(x=w5535, y=w5531) -> (x >= y?=w5536:bool)
                      n2949 = Add(x=w5555, y=w5543) -> (x+y=w5553:i32[])
                      n2950 = Multiply(x=w5486, y=w5481) -> (x*y=w5487:i32[])
                      n2951 = Index Array(array=w5544, index (col)=w5484) -> (element=w5547:u8[])  [unwired: 1 in]
                      n2952 = Increment(x=w5481) -> (x+1=w5554:i32)
                      n2953 = Add(x=w5487, y=w5480) -> (x+y=w5489:i32[])
                      n2954 = Multiply(x=w5547, y=w5481) -> (x*y=w5548:i32[])
                      n2955 = Divide(x=w5553, y=w5554) -> (x/y=w5552:dbl[])
                      n2956 = Increment(x=w5481) -> (x+1=w5488:i32)
                      n2957 = Add(x=w5548, y=w5542) -> (x+y=w5550:i32[])
                      n2958 = Increment(x=w5481) -> (x+1=w5549:i32)
                      n2959 = Divide(x=w5489, y=w5488) -> (x/y=w5490:dbl[])
                      n2960 = Replace Array Subset(array=w5546, new element=w5552, index (col)=w5484) -> (w5545:u8[][])  [unwired: 1 in]
                      n2961 = Divide(x=w5550, y=w5549) -> (x/y=w5551:dbl[])
                      n2962 = Replace Array Subset(array=w5485, new element=w5490, index (col)=w5484) -> (w5483:u8[][])  [unwired: 1 in]
                      n2963 = Replace Array Subset(array=w5544, new element=w5551, index (col)=w5484) -> (w5541:u8[][])  [unwired: 1 in]
                      n2964 = case shown="True" w5536 {
                        tunnel: [w5663 w5666] -> w5562
                        tunnel: w5563 -> [w5663 _]
                        tunnel: w5545 -> [_ w5665]
                        tunnel: w5541 -> [_ w5664]
                        frame False {
                        }
                        frame True {
                          n2965 = local write "Image 1"(w5665) -> ()
                          n2966 = local write "Image 2"(w5664) -> ()
                          n2967 = Tick Count (ms)() -> (millisecond timer value=w5666:u32)
                        }
                      }
                    }
                    n2968 = Or(x=w5375, y=w5376) -> (x .or. y?=w5347:bool)
                    n2969 = local write "#"(w5373) -> ()
                    n2970 = Compound Arithmetic op=OR(w5343, w5345, w5344, w5347, w5346) -> (w5328:bool)
                    n2971 = Or(x=w5328, y=w5329) -> (x .or. y?=w5327:bool)
                    n2972 = case shown="True" w5327 {
